vi "NUMDEN.vi"(3 "Retardo":dbl, 4 "DENOMINADOR":dbl[](array[numeric]), 5 "NUMERADOR":dbl[](array[numeric])) -> (0 "den":string, 1 "expo":string, 2 "num":string)   [LabVIEW 2019]
panel:
  # "Y(S)"
  # "="
  # "U(S)"
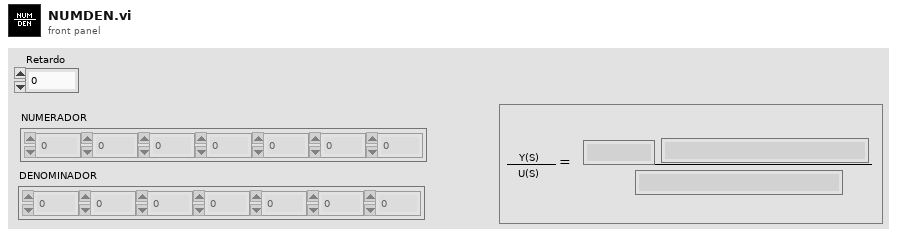
[diagram p1: front panel]
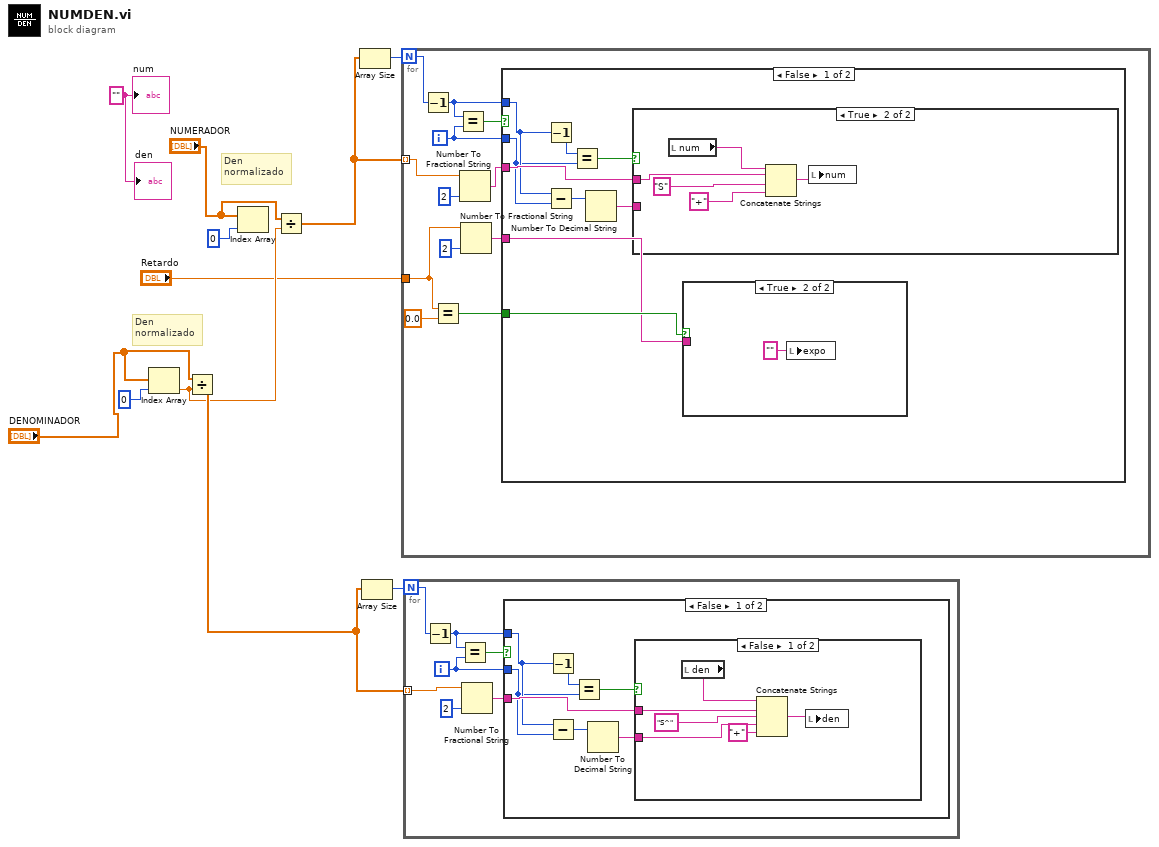
[diagram p0: block diagram]
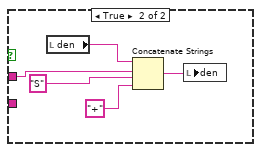
[diagram p2: hidden frame]
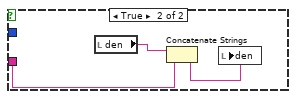
[diagram p3: hidden frame]
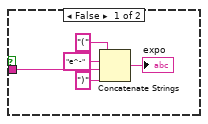
[diagram p4: hidden frame]
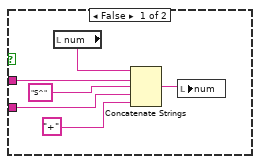
[diagram p5: hidden frame]
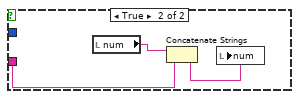
[diagram p6: hidden frame]
diagram:
  w10 = "" ("num")
  # "Den\nnormalizado"
  # "Den\nnormalizado"
  n1 = Index Array(array="DENOMINADOR", index=0) -> (element=w4:dbl)
  n2 = Divide(x="DENOMINADOR", y=w4) -> (x/y=w6:dbl[])
  n3 = Index Array(array="NUMERADOR", index=0) -> ()  [unwired: 1 out]
  n4 = Divide(x="NUMERADOR", y=w4) -> (x/y=w2:dbl[])
  n5 = Array Size(array=w2) -> (size(s)=w11:i32)
  n6 = Array Size(array=w6) -> (size(s)=w9:i32)
  n7 = for {
    N: w11 -> [w21]
    tunnel: w2 -> [w18] mode=indexing
    tunnel: "Retardo" -> [w14]
    i -> [w22]
    n8 = Decrement(x=w21) -> (x-1=w20:i32)
    n9 = Equal?(x=w14, y=0.0) -> (x = y?=w12:bool)
    n10 = Equal?(x=w20, y=w22) -> (x = y?=w23:bool)
    n11 = Number To Fractional String(number=w18, precision (6)=i16 2) -> (F-format string=w19:string)  [unwired: 2 in]
    n12 = Number To Fractional String(number=w14, precision (6)=i16 2) -> (F-format string=w15:string)  [unwired: 2 in]
    n13 = case shown="False" w23 {
      tunnel: w19 -> [w30 w51]
      tunnel: w20 -> [w29 _]
      tunnel: w22 -> [w28 _]
      tunnel: w15 -> [w24 _]
      tunnel: w12 -> [w25 _]
      frame False {
        n14 = Decrement(x=w29) -> (x-1=w31:i32)
        n15 = Subtract(x=w29, y=w28) -> (x-y=w27:i32)
        n16 = Equal?(x=w31, y=w28) -> (x = y?=w32:bool)
        n17 = Number To Decimal String(number=w27) -> (decimal integer string=w26:string)  [unwired: 1 in]
        n18 = case shown="True" w32 {
          tunnel: w30 -> [w43 w48]
          tunnel: w26 -> [w39 _]
          frame False {
            n19 = local read "num"() -> (w44:string)
            n20 = Concatenate Strings(w44, w43, "S^" ("string"), w39, "+" ("string")) -> (w40:string)
            n21 = local write "num"(w40) -> ()
          }
          frame True {
            n22 = local read "num"() -> (w49:string)
            n23 = Concatenate Strings(w49, w48, "S" ("string"), "+" ("string")) -> (w45:string)
            n24 = local write "num"(w45) -> ()
          }
        }
        n25 = case shown="True" w25 {
          tunnel: w24 -> [w33 _]
          frame False {
            n26 = Concatenate Strings("(" ("string"), "e^-" ("string"), w33, ")" ("string")) -> (→"expo":string)
          }
          frame True {
            n27 = local write "expo"("" ("expo")) -> ()
          }
        }
      }
      frame True {
        n28 = local read "num"() -> (w52:string)
        n29 = Concatenate Strings(w52, w51) -> (w50:string)
        n30 = local write "num"(w50) -> ()
      }
    }
  }
  n31 = for {
    N: w9 -> [w55]
    tunnel: w6 -> [w58] mode=indexing
    i -> [w56]
    n32 = Decrement(x=w55) -> (x-1=w54:i32)
    n33 = Equal?(x=w54, y=w56) -> (x = y?=w59:bool)
    n34 = Number To Fractional String(number=w58, precision (6)=i16 2) -> (F-format string=w57:string)  [unwired: 2 in]
    n35 = case shown="False" w59 {
      tunnel: w57 -> [w64 w79]
      tunnel: w54 -> [w63 _]
      tunnel: w56 -> [w62 _]
      frame False {
        n36 = Decrement(x=w63) -> (x-1=w65:i32)
        n37 = Subtract(x=w63, y=w62) -> (x-y=w61:i32)
        n38 = Equal?(x=w65, y=w62) -> (x = y?=w66:bool)
        n39 = Number To Decimal String(number=w61) -> (decimal integer string=w60:string)  [unwired: 1 in]
        n40 = case shown="False" w66 {
          tunnel: w64 -> [w71 w76]
          tunnel: w60 -> [w68 _]
          frame False {
            n41 = local read "den"() -> (w72:string)
            n42 = Concatenate Strings(w72, w71, "S^" ("string"), w68, "+" ("string")) -> (w69:string)
            n43 = local write "den"(w69) -> ()
          }
          frame True {
            n44 = local read "den"() -> (w77:string)
            n45 = Concatenate Strings(w77, w76, "S" ("string"), "+" ("string")) -> (w73:string)
            n46 = local write "den"(w73) -> ()
          }
        }
      }
      frame True {
        n47 = local read "den"() -> (w80:string)
        n48 = Concatenate Strings(w80, w79) -> (w78:string)
        n49 = local write "den"(w78) -> ()
      }
    }
  }
  "num" <- w10
  "den" <- w10
